vi "getWeatherData.vi"(8 "error in (no error)":errorcluster, 11 "WeatherData in":refnum<class "WeatherData.lvclass">) -> (0 "error out":errorcluster, 2 "WeatherData":T1, 3 "WeatherData out":refnum<class "WeatherData.lvclass">)   [LabVIEW 2018, in "WeatherData.lvclass"]
uses:
  WeatherData.lvclass
  WeatherData.lvclass/WeatherData.ctl
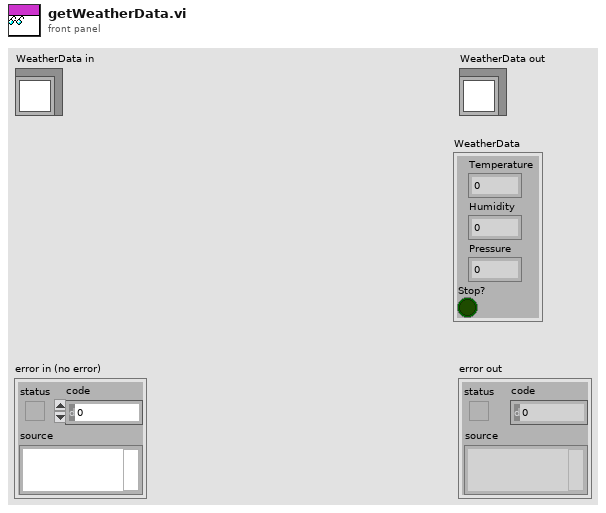
[diagram p1: front panel]
types:
  T1 = cluster{"Temperature":dbl, "Humidity":dbl, "Pressure":dbl, "Stop?":bool}
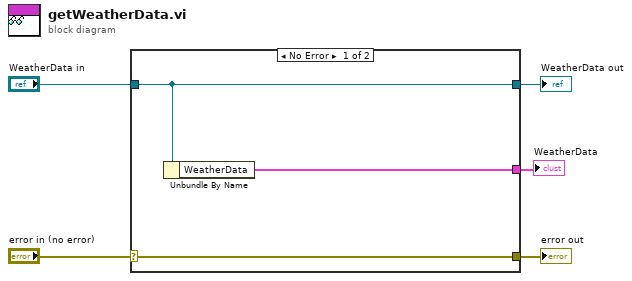
[diagram p0: block diagram]
diagram:
  n1 = case shown="No Error" "error in (no error)" {
    selector: "error in (no error)" -> [w8 w9]
    tunnel: [w8 w9] -> w4
    tunnel: [w7 w10] -> w2
    tunnel: "WeatherData in" -> [w7 w10]
    tunnel: [w6 _] -> w1
    frame No Error {
      n2 = Unbundle By Name(w7) -> ("WeatherData"=w6:T1)
    }
    frame Error {
    }
  }
  "error out" <- w4
  "WeatherData out" <- w2
  "WeatherData" <- w1
